vi "TDK电流加载及换向回读.vi"(0 "仪器实例 in":T1, 2 "输入电流":dbl, 3 "Delay Time (s)":dbl=0.1 caption="延迟时间(s)", 5 "error in":errorcluster) -> (14 "仪器实例 out":T1, 16 "实际电流":dbl, 19 "error out":errorcluster)   [LabVIEW 2020]
uses:
  F:/F020/S7_1200 control/HslCommunication.dll
  S7_1200 control/HslCommunication.dll
  <instrlib>/Keithley 27XX/Public/Data/Read Single Point.vi
  S7_1200 control/S7_1200 WriteBools.vi
  <instrlib>/Keithley 27XX/Keithley 27XX.lvlib
  S7_1200 control/S7_1200 control.lvlib
  <instrlib>/TDK-Lambda G Series/TDK-Lambda G Series.lvlib
panel:
  # "TDK 电流加载及换向"
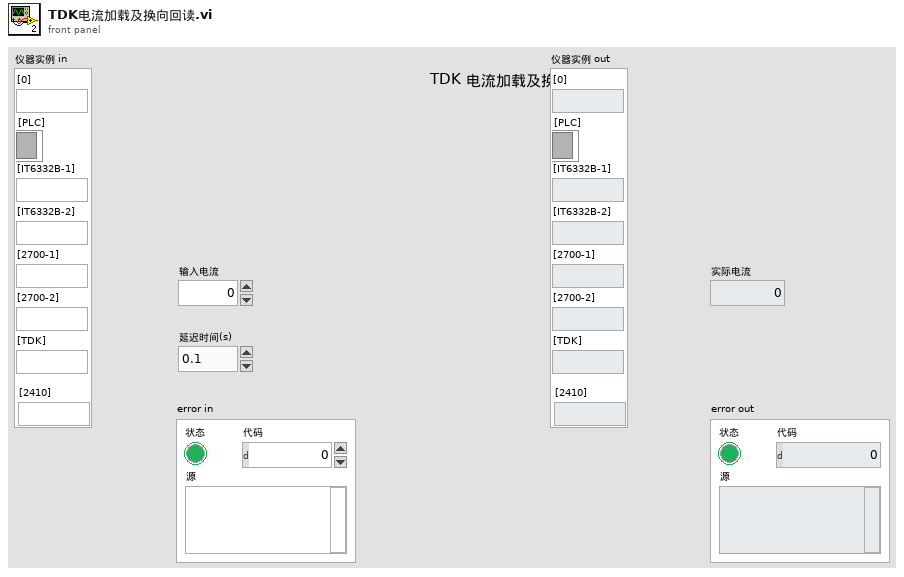
[diagram p1: front panel]
types:
  T1 = typedef "仪器实例.ctl" = cluster{"[0]":string, "[PLC]":refnum<k24>, "[IT6332B-1]":string, "[IT6332B-2]":string, "[2700-1]":string, "[2700-2]":string, "[TDK]":string, "[2410]":string}
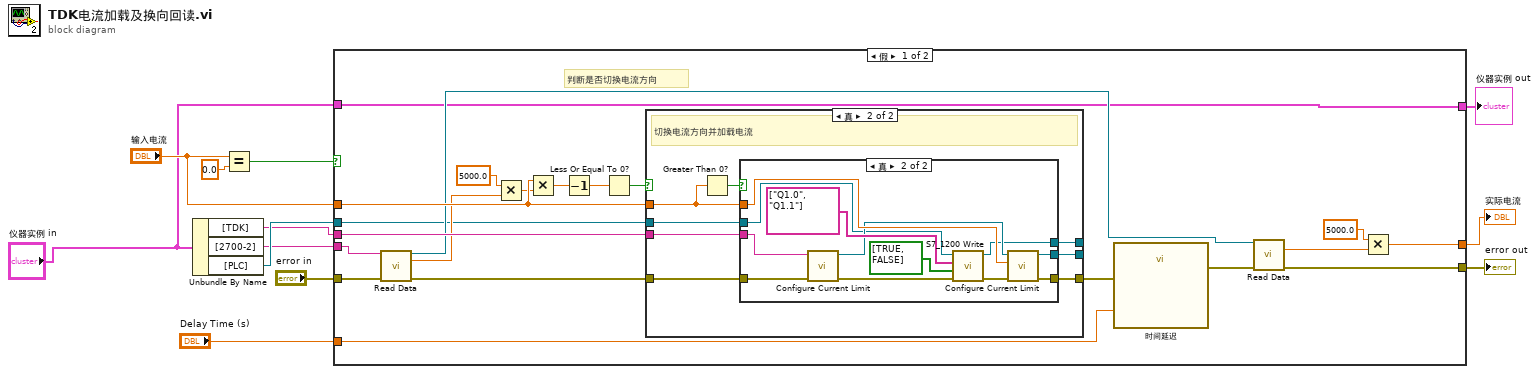
[diagram p0: block diagram]
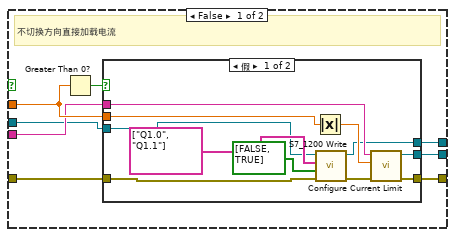
[diagram p2: hidden frame]
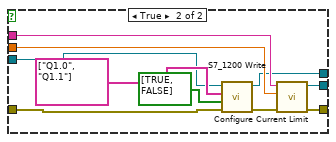
[diagram p3: hidden frame]
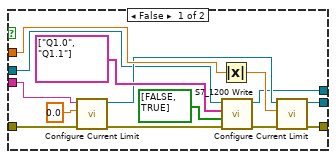
[diagram p4: hidden frame]
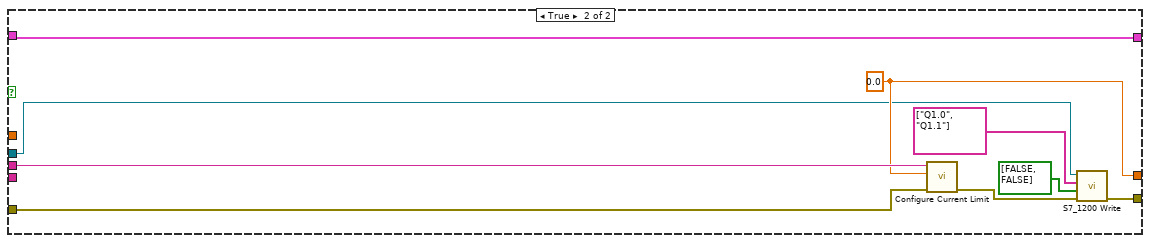
[diagram p5: hidden frame]
diagram:
  n1 = Unbundle By Name("仪器实例 in") -> ("[TDK]"=w3:string, "[2700-2]"=w4:string, "[PLC]"=w5:refnum<k24>)
  n2 = Equal?(x="输入电流", y=0.0) -> (x = y?=w8:bool)
  n3 = case shown="假" w8 {
    tunnel: w3 -> [w30 w103]
    tunnel: [w21 w99] -> w6
    tunnel: "Delay Time (s)" -> [w28 _]
    tunnel: "error in" -> [w25 w100]
    tunnel: w4 -> [w26 _]
    tunnel: "输入电流" -> [w27 _]
    tunnel: [w15 w101] -> w7
    tunnel: w5 -> [w14 w98]
    tunnel: [w13 w97] -> w1
    tunnel: "仪器实例 in" -> [w13 w97]
    frame False {
      # "判断是否切换电流方向"
      n4 = call-poly <instrlib>:"Read Data.vi"("VISA resource name"=w26, "error in (no error)"=w25) -> ("VISA resource name out"=w23:refnum<visa-resource-name>, "Measurement Data"=w20:dbl, "error out"=w24:errorcluster)  [unwired: 11 in]
      n5 = Multiply(x=5000.0, y=w20) -> (x*y=w18:dbl)
      n6 = Multiply(x=w27, y=w18) -> (x*y=w32:dbl)
      n7 = Decrement(x=w32) -> (x-1=w31:dbl)
      n8 = Less Or Equal To 0?(x=w31) -> (x <= 0?=w33:bool)
      n9 = case shown="真" w33 {
        tunnel: w27 -> [w40 w70]
        tunnel: w24 -> [w37 w66]
        tunnel: w30 -> [w39 w68]
        tunnel: [w38 w67] -> w29
        tunnel: [w36 w65] -> _
        tunnel: w14 -> [w35 w64]
        tunnel: [w34 w63] -> _
        frame False {
          # "不切换方向直接加载电流"
          n10 = Greater Than 0?(x=w40) -> (x > 0?=w41:bool)
          n11 = case shown="假" w41 {
            tunnel: w40 -> [w52 w60]
            tunnel: w39 -> [w43 w59]
            tunnel: [w51 w57] -> w38
            tunnel: w37 -> [w47 w55]
            tunnel: [w50 w56] -> w36
            tunnel: w35 -> [w45 w54]
            tunnel: [w42 w53] -> w34
            frame False {
              n12 = Absolute Value(x=w52) -> (abs(x)=w44:dbl)
              n13 = call-poly "S7_1200 Write.vi"("错误输入（无错误）"=w47, "values"=bool[] [FALSE, TRUE], "addresses"=string[] ["Q1.0", "Q1.1"], "引用"=w45) -> ("错误输出"=w49:errorcluster, "引用输出"=w42:refnum<k24>)  [unwired: 2 in]
              n14 = call <instrlib>:"Configure Current Limit.vi"("error in (no error)"=w49, "Current Limit (0A)"=w44, "VISA resource name"=w43) -> ("error out"=w51:errorcluster, "VISA resource name out"=w50:refnum<visa-resource-name>)  [unwired: 7 in]
            }
            frame True {
              n15 = call-poly "S7_1200 Write.vi"("错误输入（无错误）"=w55, "values"=bool[] [TRUE, FALSE] ("coil values"), "addresses"=string[] ["Q1.0", "Q1.1"], "引用"=w54) -> ("错误输出"=w58:errorcluster, "引用输出"=w53:refnum<k24>)  [unwired: 2 in]
              n16 = call <instrlib>:"Configure Current Limit.vi"("error in (no error)"=w58, "Current Limit (0A)"=w60, "VISA resource name"=w59) -> ("error out"=w57:errorcluster, "VISA resource name out"=w56:refnum<visa-resource-name>)  [unwired: 7 in]
            }
          }
        }
        frame True {
          # "切换电流方向并加载电流"
          n17 = Greater Than 0?(x=w70) -> (x > 0?=w69:bool)
          n18 = case shown="真" w69 {
            tunnel: w70 -> [w84 w94]
            tunnel: w68 -> [w81 w88]
            tunnel: [w76 w91] -> w67
            tunnel: w66 -> [w79 w90]
            tunnel: [w73 w92] -> w65
            tunnel: w64 -> [w72 w86]
            tunnel: [w71 w85] -> w63
            frame False {
              n19 = call <instrlib>:"Configure Current Limit.vi"("error in (no error)"=w79, "Current Limit (0A)"=0.0 ("Curr(0)"), "VISA resource name"=w81) -> ("error out"=w78:errorcluster, "VISA resource name out"=w74:refnum<visa-resource-name>)  [unwired: 7 in]
              n20 = Absolute Value(x=w84) -> (abs(x)=w75:dbl)
              n21 = call-poly "S7_1200 Write.vi"("错误输入（无错误）"=w78, "values"=bool[] [FALSE, TRUE], "addresses"=string[] ["Q1.0", "Q1.1"], "引用"=w72) -> ("错误输出"=w77:errorcluster, "引用输出"=w71:refnum<k24>)  [unwired: 2 in]
              n22 = call <instrlib>:"Configure Current Limit.vi"("error in (no error)"=w77, "Current Limit (0A)"=w75, "VISA resource name"=w74) -> ("error out"=w76:errorcluster, "VISA resource name out"=w73:refnum<visa-resource-name>)  [unwired: 7 in]
            }
            frame True {
              n23 = call <instrlib>:"Configure Current Limit.vi"("error in (no error)"=w90, "VISA resource name"=w88) -> ("error out"=w89:errorcluster, "VISA resource name out"=w87:refnum<visa-resource-name>)  [unwired: 8 in]
              n24 = call-poly "S7_1200 Write.vi"("错误输入（无错误）"=w89, "values"=bool[] [TRUE, FALSE] ("coil values"), "addresses"=string[] ["Q1.0", "Q1.1"], "引用"=w86) -> ("错误输出"=w93:errorcluster, "引用输出"=w85:refnum<k24>)  [unwired: 2 in]
              n25 = call <instrlib>:"Configure Current Limit.vi"("error in (no error)"=w93, "Current Limit (0A)"=w94, "VISA resource name"=w87) -> ("error out"=w91:errorcluster, "VISA resource name out"=w92:refnum<visa-resource-name>)  [unwired: 7 in]
            }
          }
        }
      }
      n26 = call "时间延迟"("error in (no error)"=w29, "Delay Time (s)"=w28) -> ("error out"=w22:errorcluster)  [unwired: 9 in]
      n27 = call-poly <instrlib>:"Read Data.vi"("VISA resource name"=w23, "error in (no error)"=w22) -> ("Measurement Data"=w17:dbl, "error out"=w21:errorcluster)  [unwired: 11 in, 1 out]
      n28 = Multiply(x=5000.0, y=w17) -> (x*y=w15:dbl)
    }
    frame True {
      w101 = 0.0 ("Curr(0)")
      n29 = call <instrlib>:"Configure Current Limit.vi"("error in (no error)"=w100, "Current Limit (0A)"=w101, "VISA resource name"=w103) -> ("error out"=w102:errorcluster)  [unwired: 7 in, 1 out]
      n30 = call-poly "S7_1200 Write.vi"("错误输入（无错误）"=w102, "values"=bool[] [FALSE, FALSE], "addresses"=string[] ["Q1.0", "Q1.1"], "引用"=w98) -> ("错误输出"=w99:errorcluster)  [unwired: 2 in, 1 out]
    }
  }
  "error out" <- w6
  "实际电流" <- w7
  "仪器实例 out" <- w1
